vi "Configure Trigger (Width).vi"(0 "VISA resource name":refnum<visa-resource-name>, 1 "Width Condition (0: Within)":u16(ring) items=["Within", "Outside"], 2 "Width  (1.5E-9)":dbl=1.5e-09, 5 "Trigger Source (1: Channel 1)":u16(ring)=1 items=["Channel 1"=1, "Channel 2"=2, "Channel 3"=3, "Channel 4"=4, "Digital 0"=13, "Digital 1"=14, "Digital 2"=15, "Digital 3"=16, "Digital 4"=17, "Digital 5"=18, "Digital 6"=19, "Digital 7"=20, "Digital 8"=21, "Digital 9"=22, "Digital 10"=23, "Digital 11"=24, "Digital 12"=25, "Digital 13"=26, "Digital 14"=27, "Digital 15"=28], 7 "Trigger Level  (0 V)":dbl, 9 "Width Polarity (0: Positive)":u16(ring) items=["Positive", "Negative"], 11 "error in (no error)":errorcluster) -> (4 "VISA resource name out":refnum<visa-resource-name>, 15 "error out":errorcluster)   [LabVIEW 2012, in "Agilent 8000 Series.lvlib"]
doc: "Configures the width trigger. A width trigger occurs when the oscilloscope detects a positive or negative pulse with a width between, or optionally outside, the width thresholds. You specify the width thresholds with the Width Low Threshold and Width High Threshold parameters. You specify whether the oscilloscope triggers on pulse widths that are within or outside the width thresholds with the Width Condition parameter. You specify the polarity of the pulse with the Width Polarity parameter. The trigger does not actually occur until the edge of a pulse that corresponds to the Width Low Threshold, Width High Threshold, Width Condition, and Width Polarity crosses the threshold you specify in the Trigger Level parameter."
uses:
  Agilent 8000 Series.lvlib
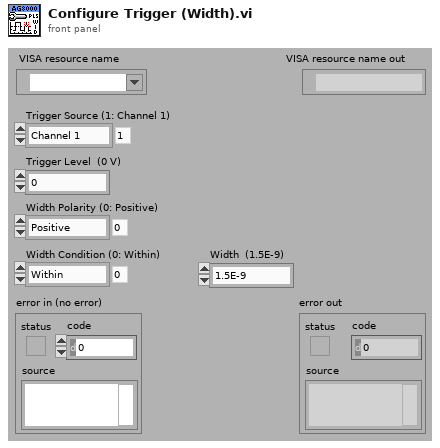
[diagram p1: front panel]
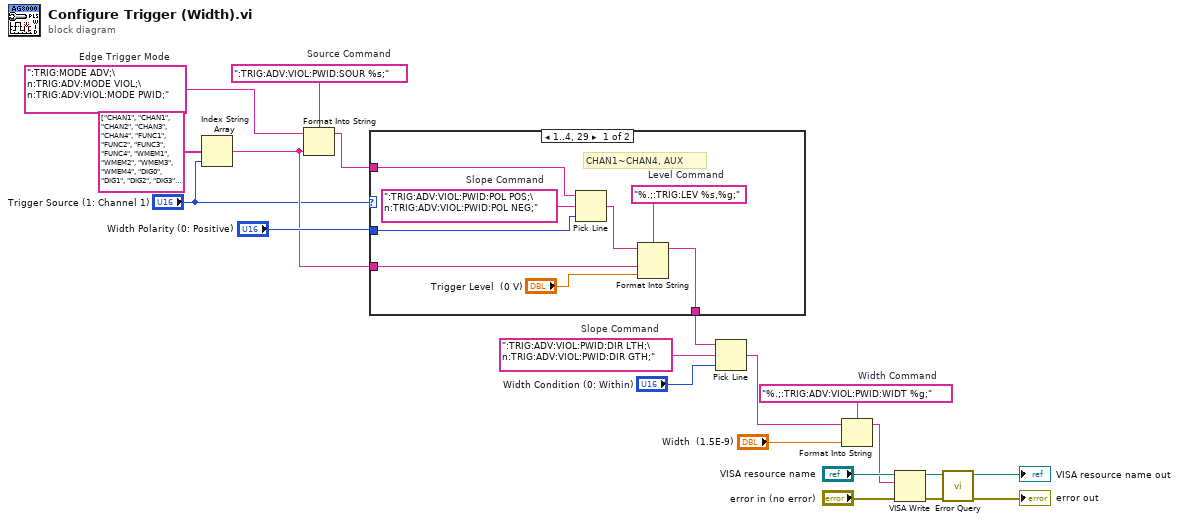
[diagram p0: block diagram]
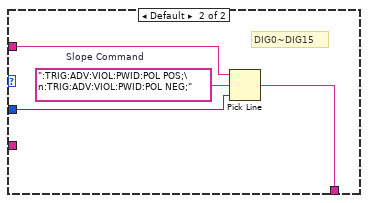
[diagram p2: hidden frame]
diagram:
  w3 = "%.;:TRIG:ADV:VIOL:PWID:WIDT %g;"  # Width Command
  w6 = ":TRIG:ADV:VIOL:PWID:DIR LTH;\n:TRIG:ADV:VIOL:PWID:DIR GTH;"  # Slope Command
  w13 = ":TRIG:ADV:VIOL:PWID:SOUR %s;"  # Source Command
  w12 = ":TRIG:MODE ADV;\n:TRIG:ADV:MODE VIOL;\n:TRIG:ADV:VIOL:MODE PWID;"  # Edge Trigger Mode
  n1 = Index String Array(1:"Trigger Source (1: Channel 1)", 2:string[] ["CHAN1", "CHAN1", "CHAN2", "CHAN3", "CHAN4", "FUNC1", "FUNC2", "FUNC3", "FUNC4", "WMEM1", "WMEM2", "WMEM3", "WMEM4", "DIG0", "DIG1", "DIG2", "DIG3", "DIG4", "DIG5", "DIG6", "DIG7", "DIG8", "DIG9", "DIG10", "DIG11", "DIG12", "DIG13", "DIG14", "DIG15", "AUX", "LINE"]) -> (0:w9:string)  [unwired: 1 in]
  n2 = Format Into String(format string=w13, initial string=w12, w9) -> (resulting string=w11:string)  [unwired: 1 in, 1 out]
  n3 = case shown="1..4, 29" "Trigger Source (1: Channel 1)" {
    tunnel: [w27 w29] -> w5
    tunnel: "Width Polarity (0: Positive)" -> [w24 w31]
    tunnel: w11 -> [w25 w30]
    tunnel: w9 -> [w22 _]
    frame 1..4, 29 {
      w26 = ":TRIG:ADV:VIOL:PWID:POL POS;\n:TRIG:ADV:VIOL:PWID:POL NEG;"  # Slope Command
      w28 = "%.;:TRIG:LEV %s,%g;"  # Level Command
      # "CHAN1~CHAN4, AUX"
      n4 = Pick Line(string ("")=w25, multi-line string=w26, line index=w24) -> (output string=w23:string)
      n5 = Format Into String(format string=w28, initial string=w23, w22, "Trigger Level  (0 V)") -> (resulting string=w27:string)  [unwired: 1 in, 1 out]
    }
    frame Default {
      w32 = ":TRIG:ADV:VIOL:PWID:POL POS;\n:TRIG:ADV:VIOL:PWID:POL NEG;"  # Slope Command
      # "DIG0~DIG15"
      n6 = Pick Line(string ("")=w30, multi-line string=w32, line index=w31) -> (output string=w29:string)
    }
  }
  n7 = Pick Line(string ("")=w5, multi-line string=w6, line index="Width Condition (0: Within)") -> (output string=w2:string)
  n8 = Format Into String(format string=w3, initial string=w2, "Width  (1.5E-9)") -> (resulting string=w1:string)  [unwired: 1 in, 1 out]
  n9 = VISA Write(VISA resource name="VISA resource name", write buffer=w1, error in (no error)="error in (no error)") -> (VISA resource name out=w16:refnum<visa-resource-name>, error out=w15:errorcluster)  [unwired: 1 out]
  n10 = call "Error Query.vi"("error in (no error)"=w15, "VISA resource name"=w16) -> ("error out"=→"error out":errorcluster, "VISA resource name out"=→"VISA resource name out":refnum<visa-resource-name>)  [unwired: 6 in, 2 out]
